vi "Labview.vi"() -> ()   [LabVIEW 2013]
panel:
  out "Array 7":bool[](array[boolean])
  out "Array 6":bool[](array[boolean])
  out "Boolean 7":bool
  out "Boolean 6":bool
  out "Array 5":bool[](array[boolean])
  out "Array 4":bool[](array[boolean])
  out "Array 3":bool[](array[boolean])
  out "Array 2":bool[](array[boolean])
  out "Boolean 5":bool
  out "Boolean 4":bool
  out "Boolean 3":bool
  out "Boolean 2":bool
  out "Boolean":bool
  out "Array 1":bool[](array[boolean])
  in  "string":string
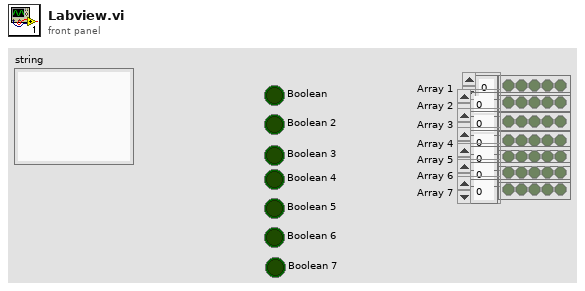
[diagram p1: front panel]
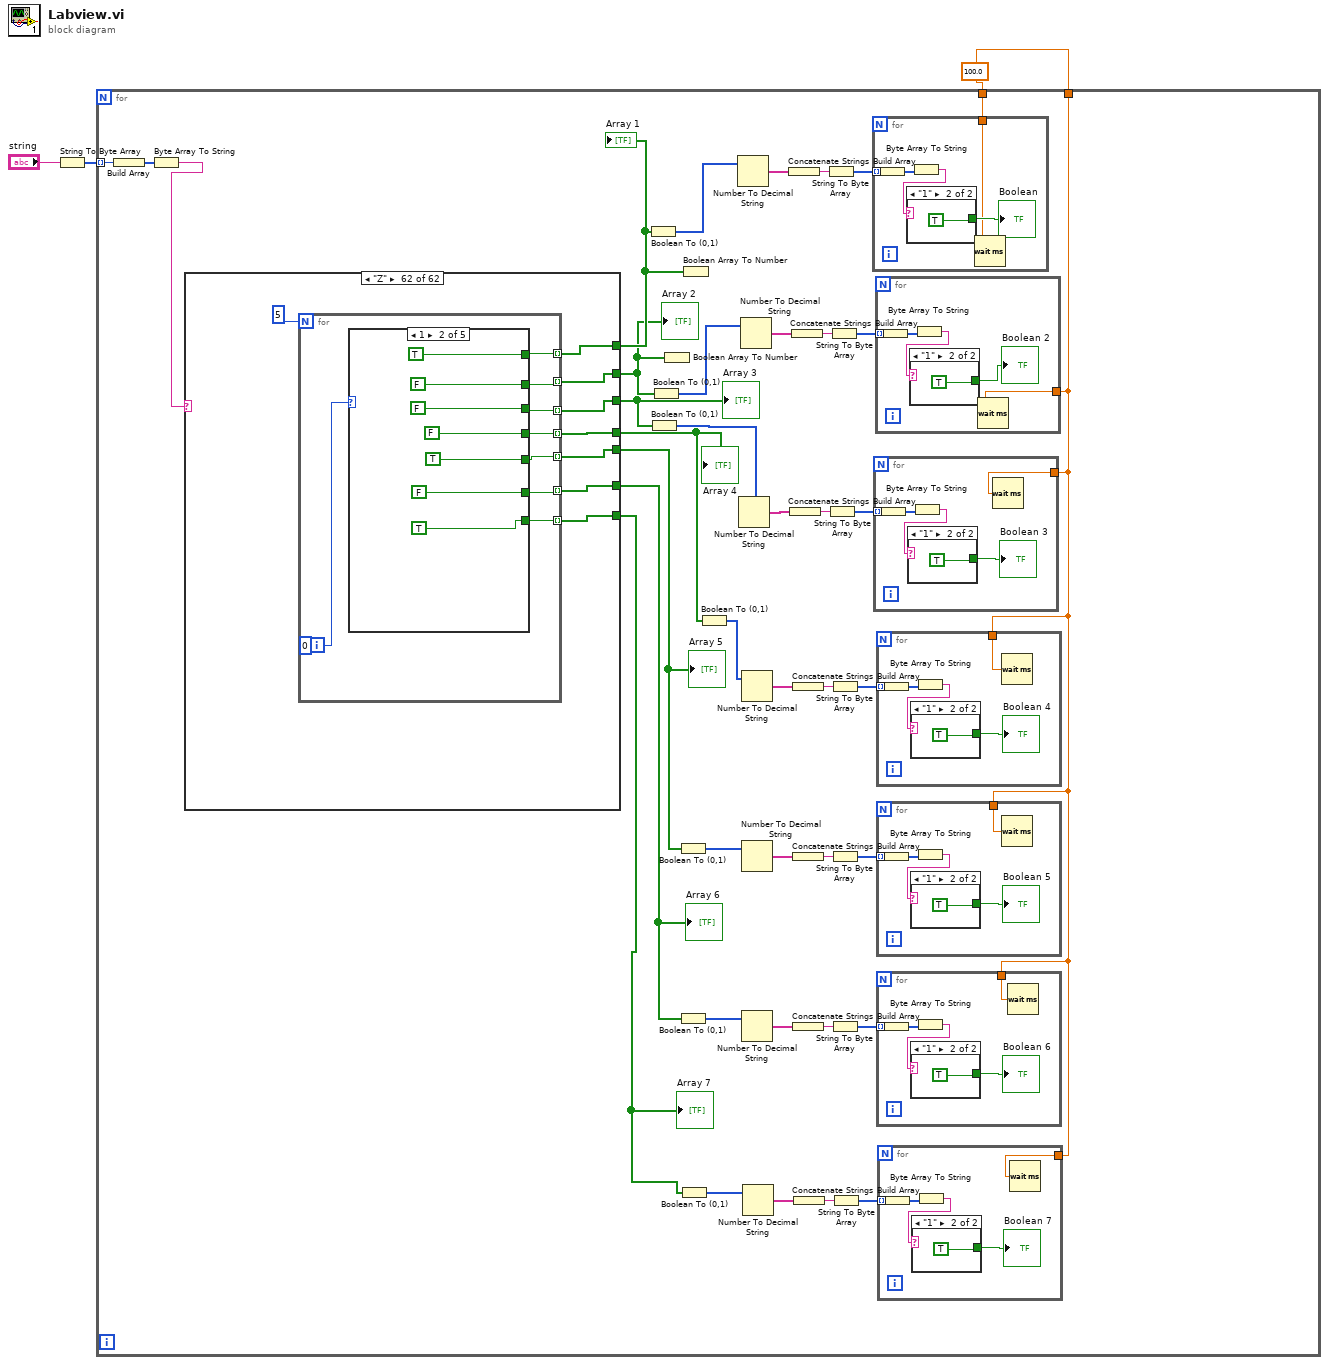
[diagram p0: block diagram]
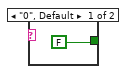
[diagram p2: hidden frame]
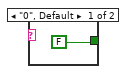
[diagram p3: hidden frame]
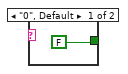
[diagram p4: hidden frame]
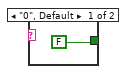
[diagram p5: hidden frame]
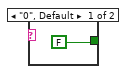
[diagram p6: hidden frame]
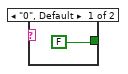
[diagram p7: hidden frame]
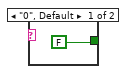
[diagram p8: hidden frame]
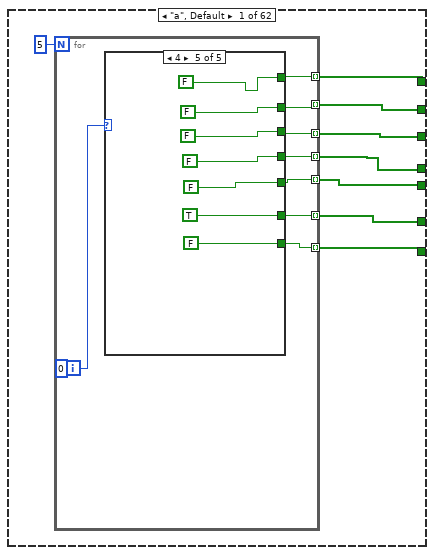
[diagram p9: hidden frame]
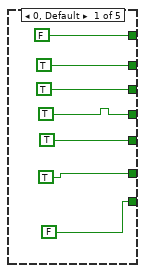
[diagram p10: hidden frame]
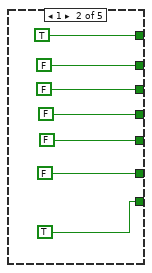
[diagram p11: hidden frame]
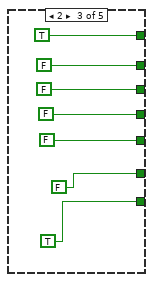
[diagram p12: hidden frame]
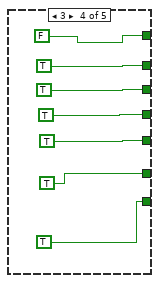
[diagram p13: hidden frame]
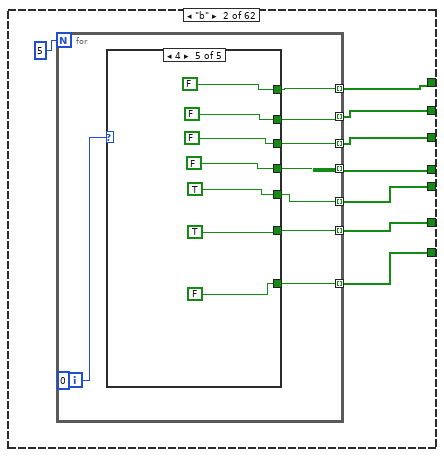
[diagram p14: hidden frame]
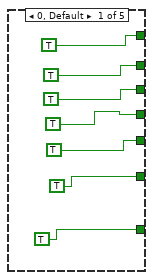
[diagram p15: hidden frame]
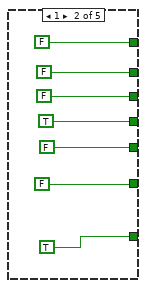
[diagram p16: hidden frame]
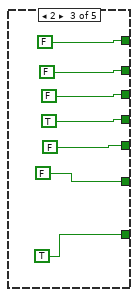
[diagram p17: hidden frame]
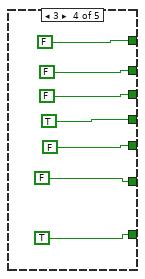
[diagram p18: hidden frame]
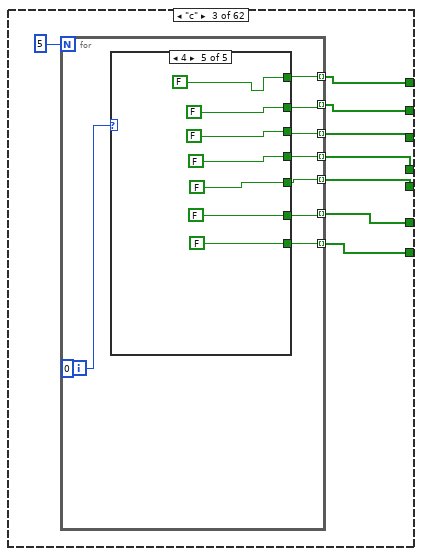
[diagram p19: hidden frame]
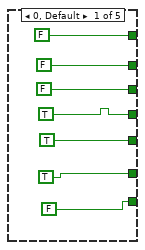
[diagram p20: hidden frame]
diagram:
  w1 = 100.0
  n1 = String To Byte Array(string="string") -> (unsigned byte array=w3:u8[])
  n2 = for {
    tunnel: w3 -> [w43] mode=indexing
    tunnel: w1 -> [w5]
    tunnel: w1 -> [w4]
    n3 = Build Array(w43) -> (w42:u8[])
    n4 = Byte Array To String(unsigned byte array=w42) -> (string=w41:string)
    n5 = case shown="\"Z\"" w41 {
      tunnel: [w99 w146 w201 w252 w303 w354 w405 w456 w507 w558 w609 w660 w711 w762 w813 w864 w915 w966 w1017 w1068 w1119 w1170 w1221 w1272 w1323 w1374 w1425 w1476 w1527 w1578 w1629 w1680 w1731 w1782 w1833 w1884 w1935 w1986 w2037 w2088 w2139 w2190 w2241 w2292 w2343 w2394 w2445 w2496 w2547 w2598 w2649 w2700 w2751 w2802 w2853 w2904 w2955 w3006 w3057 w3108 w3159 w3210] -> w18
      tunnel: [w98 w150 w200 w251 w302 w353 w404 w455 w506 w557 w608 w659 w710 w761 w812 w863 w914 w965 w1016 w1067 w1118 w1169 w1220 w1271 w1322 w1373 w1424 w1475 w1526 w1577 w1628 w1679 w1730 w1781 w1832 w1883 w1934 w1985 w2036 w2087 w2138 w2189 w2240 w2291 w2342 w2393 w2444 w2495 w2546 w2597 w2648 w2699 w2750 w2801 w2852 w2903 w2954 w3005 w3056 w3107 w3158 w3209] -> w17
      tunnel: [w97 w149 w199 w250 w301 w352 w403 w454 w505 w556 w607 w658 w709 w760 w811 w862 w913 w964 w1015 w1066 w1117 w1168 w1219 w1270 w1321 w1372 w1423 w1474 w1525 w1576 w1627 w1678 w1729 w1780 w1831 w1882 w1933 w1984 w2035 w2086 w2137 w2188 w2239 w2290 w2341 w2392 w2443 w2494 w2545 w2596 w2647 w2698 w2749 w2800 w2851 w2902 w2953 w3004 w3055 w3106 w3157 w3208] -> w29
      tunnel: [w96 w148 w198 w249 w300 w351 w402 w453 w504 w555 w606 w657 w708 w759 w810 w861 w912 w963 w1014 w1065 w1116 w1167 w1218 w1269 w1320 w1371 w1422 w1473 w1524 w1575 w1626 w1677 w1728 w1779 w1830 w1881 w1932 w1983 w2034 w2085 w2136 w2187 w2238 w2289 w2340 w2391 w2442 w2493 w2544 w2595 w2646 w2697 w2748 w2799 w2850 w2901 w2952 w3003 w3054 w3105 w3156 w3207] -> w24
      tunnel: [w95 w147 w197 w248 w299 w350 w401 w452 w503 w554 w605 w656 w707 w758 w809 w860 w911 w962 w1013 w1064 w1115 w1166 w1217 w1268 w1319 w1370 w1421 w1472 w1523 w1574 w1625 w1676 w1727 w1778 w1829 w1880 w1931 w1982 w2033 w2084 w2135 w2186 w2237 w2288 w2339 w2390 w2441 w2492 w2543 w2594 w2645 w2696 w2747 w2798 w2849 w2900 w2951 w3002 w3053 w3104 w3155 w3206] -> w16
      tunnel: [w94 w145 w196 w247 w298 w349 w400 w451 w502 w553 w604 w655 w706 w757 w808 w859 w910 w961 w1012 w1063 w1114 w1165 w1216 w1267 w1318 w1369 w1420 w1471 w1522 w1573 w1624 w1675 w1726 w1777 w1828 w1879 w1930 w1981 w2032 w2083 w2134 w2185 w2236 w2287 w2338 w2389 w2440 w2491 w2542 w2593 w2644 w2695 w2746 w2797 w2848 w2899 w2950 w3001 w3052 w3103 w3154 w3205] -> w7
      tunnel: [w93 w144 w195 w246 w297 w348 w399 w450 w501 w552 w603 w654 w705 w756 w807 w858 w909 w960 w1011 w1062 w1113 w1164 w1215 w1266 w1317 w1368 w1419 w1470 w1521 w1572 w1623 w1674 w1725 w1776 w1827 w1878 w1929 w1980 w2031 w2082 w2133 w2184 w2235 w2286 w2337 w2388 w2439 w2490 w2541 w2592 w2643 w2694 w2745 w2796 w2847 w2898 w2949 w3000 w3051 w3102 w3153 w3204] -> w6
      frame "a", Default {
        n6 = for {
          N: 5 -> [_]
          tunnel: [w107] -> w99 mode=indexing
          tunnel: [w106] -> w98 mode=indexing
          tunnel: [w105] -> w97 mode=indexing
          tunnel: [w104] -> w96 mode=indexing
          tunnel: [w103] -> w95 mode=indexing
          tunnel: [w102] -> w94 mode=indexing
          tunnel: [w101] -> w93 mode=indexing
          i -> [w108]
          (unwired) 0
          n7 = case shown="4" w108 {
            tunnel: [FALSE TRUE TRUE FALSE FALSE] -> w107
            tunnel: [TRUE FALSE FALSE TRUE FALSE] -> w106
            tunnel: [TRUE FALSE FALSE TRUE FALSE] -> w105
            tunnel: [TRUE FALSE FALSE TRUE FALSE] -> w104
            tunnel: [TRUE FALSE FALSE TRUE FALSE] -> w103
            tunnel: [TRUE FALSE FALSE TRUE TRUE] -> w102
            tunnel: [FALSE TRUE TRUE TRUE FALSE] -> w101
            frame 0, Default {
            }
            frame 1 {
            }
            frame 2 {
            }
            frame 3 {
            }
            frame 4 {
            }
          }
        }
      }
      frame "b" {
        n8 = for {
          N: 5 -> [_]
          tunnel: [w158] -> w146 mode=indexing
          tunnel: [w157] -> w150 mode=indexing
          tunnel: [w156] -> w149 mode=indexing
          tunnel: [w155] -> w148 mode=indexing
          tunnel: [w154] -> w147 mode=indexing
          tunnel: [w153] -> w145 mode=indexing
          tunnel: [w152] -> w144 mode=indexing
          i -> [w159]
          (unwired) 0
          n9 = case shown="4" w159 {
            tunnel: [TRUE FALSE FALSE FALSE FALSE] -> w158
            tunnel: [TRUE FALSE FALSE FALSE FALSE] -> w157
            tunnel: [TRUE FALSE FALSE FALSE FALSE] -> w156
            tunnel: [TRUE TRUE TRUE TRUE FALSE] -> w155
            tunnel: [TRUE FALSE FALSE FALSE TRUE] -> w154
            tunnel: [TRUE FALSE FALSE FALSE TRUE] -> w153
            tunnel: [TRUE TRUE TRUE TRUE FALSE] -> w152
            frame 0, Default {
            }
            frame 1 {
            }
            frame 2 {
            }
            frame 3 {
            }
            frame 4 {
            }
          }
        }
      }
      frame "c" {
        n10 = for {
          N: 5 -> [_]
          tunnel: [w209] -> w201 mode=indexing
          tunnel: [w208] -> w200 mode=indexing
          tunnel: [w207] -> w199 mode=indexing
          tunnel: [w206] -> w198 mode=indexing
          tunnel: [w205] -> w197 mode=indexing
          tunnel: [w204] -> w196 mode=indexing
          tunnel: [w203] -> w195 mode=indexing
          i -> [w210]
          (unwired) 0
          n11 = case shown="4" w210 {
            tunnel: [FALSE FALSE FALSE FALSE FALSE] -> w209
            tunnel: [FALSE FALSE FALSE FALSE FALSE] -> w208
            tunnel: [FALSE TRUE TRUE FALSE FALSE] -> w207
            tunnel: [TRUE FALSE FALSE TRUE FALSE] -> w206
            tunnel: [TRUE FALSE FALSE FALSE FALSE] -> w205
            tunnel: [TRUE FALSE FALSE FALSE FALSE] -> w204
            tunnel: [FALSE TRUE TRUE TRUE FALSE] -> w203
            frame 0, Default {
            }
            frame 1 {
            }
            frame 2 {
            }
            frame 3 {
            }
            frame 4 {
            }
          }
        }
      }
      frame "d" {
        n12 = for {
          N: 5 -> [_]
          tunnel: [w260] -> w252 mode=indexing
          tunnel: [w259] -> w251 mode=indexing
          tunnel: [w258] -> w250 mode=indexing
          tunnel: [w257] -> w249 mode=indexing
          tunnel: [w256] -> w248 mode=indexing
          tunnel: [w255] -> w247 mode=indexing
          tunnel: [w254] -> w246 mode=indexing
          i -> [w261]
          (unwired) 0
          n13 = case shown="0, Default" w261 {
            tunnel: [FALSE FALSE FALSE FALSE TRUE] -> w260
            tunnel: [FALSE FALSE FALSE FALSE TRUE] -> w259
            tunnel: [FALSE TRUE TRUE TRUE TRUE] -> w258
            tunnel: [TRUE FALSE FALSE FALSE TRUE] -> w257
            tunnel: [TRUE FALSE FALSE FALSE TRUE] -> w256
            tunnel: [TRUE FALSE FALSE FALSE TRUE] -> w255
            tunnel: [FALSE TRUE TRUE TRUE TRUE] -> w254
            frame 0, Default {
            }
            frame 1 {
            }
            frame 2 {
            }
            frame 3 {
            }
            frame 4 {
            }
          }
        }
      }
      frame "e" {
        n14 = for {
          N: 5 -> [_]
          tunnel: [w311] -> w303 mode=indexing
          tunnel: [w310] -> w302 mode=indexing
          tunnel: [w309] -> w301 mode=indexing
          tunnel: [w308] -> w300 mode=indexing
          tunnel: [w307] -> w299 mode=indexing
          tunnel: [w306] -> w298 mode=indexing
          tunnel: [w305] -> w297 mode=indexing
          i -> [w312]
          (unwired) 0
          n15 = case shown="0, Default" w312 {
            tunnel: [FALSE FALSE FALSE FALSE FALSE] -> w311
            tunnel: [FALSE FALSE FALSE FALSE FALSE] -> w310
            tunnel: [FALSE TRUE TRUE TRUE TRUE] -> w309
            tunnel: [TRUE FALSE FALSE FALSE TRUE] -> w308
            tunnel: [TRUE TRUE TRUE TRUE TRUE] -> w307
            tunnel: [TRUE FALSE FALSE FALSE FALSE] -> w306
            tunnel: [FALSE TRUE TRUE TRUE TRUE] -> w305
            frame 0, Default {
            }
            frame 1 {
            }
            frame 2 {
            }
            frame 3 {
            }
            frame 4 {
            }
          }
        }
      }
      frame "f" {
        n16 = for {
          N: 5 -> [_]
          tunnel: [w362] -> w354 mode=indexing
          tunnel: [w361] -> w353 mode=indexing
          tunnel: [w360] -> w352 mode=indexing
          tunnel: [w359] -> w351 mode=indexing
          tunnel: [w358] -> w350 mode=indexing
          tunnel: [w357] -> w349 mode=indexing
          tunnel: [w356] -> w348 mode=indexing
          i -> [w363]
          (unwired) 0
          n17 = case shown="0, Default" w363 {
            tunnel: [FALSE FALSE TRUE TRUE FALSE] -> w362
            tunnel: [FALSE FALSE TRUE FALSE TRUE] -> w361
            tunnel: [FALSE FALSE TRUE FALSE FALSE] -> w360
            tunnel: [FALSE TRUE TRUE TRUE FALSE] -> w359
            tunnel: [FALSE FALSE TRUE FALSE FALSE] -> w358
            tunnel: [FALSE FALSE TRUE FALSE FALSE] -> w357
            tunnel: [FALSE TRUE TRUE FALSE FALSE] -> w356
            frame 0, Default {
            }
            frame 1 {
            }
            frame 2 {
            }
            frame 3 {
            }
            frame 4 {
            }
          }
        }
      }
      frame "g" {
        n18 = for {
          N: 5 -> [_]
          tunnel: [w413] -> w405 mode=indexing
          tunnel: [w412] -> w404 mode=indexing
          tunnel: [w411] -> w403 mode=indexing
          tunnel: [w410] -> w402 mode=indexing
          tunnel: [w409] -> w401 mode=indexing
          tunnel: [w408] -> w400 mode=indexing
          tunnel: [w407] -> w399 mode=indexing
          i -> [w414]
          (unwired) 0
          n19 = case shown="0, Default" w414 {
            tunnel: [FALSE TRUE TRUE TRUE FALSE] -> w413
            tunnel: [TRUE FALSE FALSE FALSE TRUE] -> w412
            tunnel: [TRUE FALSE FALSE FALSE TRUE] -> w411
            tunnel: [FALSE FALSE TRUE TRUE TRUE] -> w410
            tunnel: [FALSE FALSE FALSE FALSE TRUE] -> w409
            tunnel: [TRUE TRUE FALSE TRUE TRUE] -> w408
            tunnel: [FALSE TRUE TRUE TRUE FALSE] -> w407
            frame 0, Default {
            }
            frame 1 {
            }
            frame 2 {
            }
            frame 3 {
            }
            frame 4 {
            }
          }
        }
      }
      frame "h" {
        n20 = for {
          N: 5 -> [_]
          tunnel: [w464] -> w456 mode=indexing
          tunnel: [w463] -> w455 mode=indexing
          tunnel: [w462] -> w454 mode=indexing
          tunnel: [w461] -> w453 mode=indexing
          tunnel: [w460] -> w452 mode=indexing
          tunnel: [w459] -> w451 mode=indexing
          tunnel: [w458] -> w450 mode=indexing
          i -> [w465]
          (unwired) 0
          n21 = case shown="0, Default" w465 {
            tunnel: [TRUE FALSE FALSE FALSE FALSE] -> w464
            tunnel: [TRUE FALSE FALSE FALSE FALSE] -> w463
            tunnel: [TRUE FALSE FALSE FALSE FALSE] -> w462
            tunnel: [TRUE TRUE TRUE TRUE FALSE] -> w461
            tunnel: [TRUE FALSE FALSE FALSE TRUE] -> w460
            tunnel: [TRUE FALSE FALSE FALSE TRUE] -> w459
            tunnel: [TRUE FALSE FALSE FALSE TRUE] -> w458
            frame 0, Default {
            }
            frame 1 {
            }
            frame 2 {
            }
            frame 3 {
            }
            frame 4 {
            }
          }
        }
      }
      frame "i" {
        n22 = for {
          N: 5 -> [_]
          tunnel: [w515] -> w507 mode=indexing
          tunnel: [w514] -> w506 mode=indexing
          tunnel: [w513] -> w505 mode=indexing
          tunnel: [w512] -> w504 mode=indexing
          tunnel: [w511] -> w503 mode=indexing
          tunnel: [w510] -> w502 mode=indexing
          tunnel: [w509] -> w501 mode=indexing
          i -> [w516]
          (unwired) 0
          n23 = case shown="4" w516 {
            tunnel: [FALSE FALSE FALSE FALSE FALSE] -> w515
            tunnel: [FALSE FALSE TRUE FALSE FALSE] -> w514
            tunnel: [FALSE FALSE FALSE FALSE FALSE] -> w513
            tunnel: [FALSE FALSE TRUE FALSE FALSE] -> w512
            tunnel: [FALSE FALSE TRUE FALSE FALSE] -> w511
            tunnel: [FALSE FALSE TRUE FALSE FALSE] -> w510
            tunnel: [FALSE FALSE TRUE FALSE FALSE] -> w509
            frame 0, Default {
            }
            frame 1 {
            }
            frame 2 {
            }
            frame 3 {
            }
            frame 4 {
            }
          }
        }
      }
      frame "j" {
        n24 = for {
          N: 5 -> [_]
          tunnel: [w566] -> w558 mode=indexing
          tunnel: [w565] -> w557 mode=indexing
          tunnel: [w564] -> w556 mode=indexing
          tunnel: [w563] -> w555 mode=indexing
          tunnel: [w562] -> w554 mode=indexing
          tunnel: [w561] -> w553 mode=indexing
          tunnel: [w560] -> w552 mode=indexing
          i -> [w567]
          (unwired) 0
          n25 = case shown="0, Default" w567 {
            tunnel: [FALSE FALSE FALSE FALSE FALSE] -> w566
            tunnel: [FALSE FALSE TRUE FALSE FALSE] -> w565
            tunnel: [FALSE FALSE FALSE FALSE FALSE] -> w564
            tunnel: [FALSE FALSE TRUE FALSE FALSE] -> w563
            tunnel: [FALSE FALSE TRUE FALSE FALSE] -> w562
            tunnel: [TRUE FALSE TRUE FALSE FALSE] -> w561
            tunnel: [FALSE TRUE TRUE FALSE FALSE] -> w560
            frame 0, Default {
            }
            frame 1 {
            }
            frame 2 {
            }
            frame 3 {
            }
            frame 4 {
            }
          }
        }
      }
      frame "k" {
        n26 = for {
          N: 5 -> [_]
          tunnel: [w617] -> w609 mode=indexing
          tunnel: [w616] -> w608 mode=indexing
          tunnel: [w615] -> w607 mode=indexing
          tunnel: [w614] -> w606 mode=indexing
          tunnel: [w613] -> w605 mode=indexing
          tunnel: [w612] -> w604 mode=indexing
          tunnel: [w611] -> w603 mode=indexing
          i -> [w618]
          (unwired) 0
          n27 = case shown="0, Default" w618 {
            tunnel: [TRUE FALSE FALSE FALSE FALSE] -> w617
            tunnel: [TRUE FALSE FALSE FALSE FALSE] -> w616
            tunnel: [TRUE FALSE FALSE TRUE FALSE] -> w615
            tunnel: [TRUE FALSE TRUE FALSE FALSE] -> w614
            tunnel: [TRUE TRUE FALSE FALSE FALSE] -> w613
            tunnel: [TRUE FALSE TRUE FALSE FALSE] -> w612
            tunnel: [TRUE FALSE FALSE TRUE FALSE] -> w611
            frame 0, Default {
            }
            frame 1 {
            }
            frame 2 {
            }
            frame 3 {
            }
            frame 4 {
            }
          }
        }
      }
      frame "l" {
        n28 = for {
          N: 5 -> [_]
          tunnel: [w668] -> w660 mode=indexing
          tunnel: [w667] -> w659 mode=indexing
          tunnel: [w666] -> w658 mode=indexing
          tunnel: [w665] -> w657 mode=indexing
          tunnel: [w664] -> w656 mode=indexing
          tunnel: [w663] -> w655 mode=indexing
          tunnel: [w662] -> w654 mode=indexing
          i -> [w669]
          (unwired) 0
          n29 = case shown="4" w669 {
            tunnel: [FALSE FALSE TRUE FALSE FALSE] -> w668
            tunnel: [FALSE FALSE TRUE FALSE FALSE] -> w667
            tunnel: [TRUE FALSE TRUE FALSE FALSE] -> w666
            tunnel: [TRUE FALSE TRUE FALSE FALSE] -> w665
            tunnel: [TRUE FALSE TRUE FALSE FALSE] -> w664
            tunnel: [TRUE FALSE TRUE FALSE FALSE] -> w663
            tunnel: [TRUE FALSE TRUE FALSE FALSE] -> w662
            frame 0, Default {
            }
            frame 1 {
            }
            frame 2 {
            }
            frame 3 {
            }
            frame 4 {
            }
          }
        }
      }
      frame "m" {
        n30 = for {
          N: 5 -> [_]
          tunnel: [w719] -> w711 mode=indexing
          tunnel: [w718] -> w710 mode=indexing
          tunnel: [w717] -> w709 mode=indexing
          tunnel: [w716] -> w708 mode=indexing
          tunnel: [w715] -> w707 mode=indexing
          tunnel: [w714] -> w706 mode=indexing
          tunnel: [w713] -> w705 mode=indexing
          i -> [w720]
          (unwired) 0
          n31 = case shown="4" w720 {
            tunnel: [FALSE FALSE FALSE FALSE FALSE] -> w719
            tunnel: [FALSE FALSE FALSE FALSE FALSE] -> w718
            tunnel: [FALSE FALSE FALSE FALSE FALSE] -> w717
            tunnel: [FALSE TRUE FALSE FALSE TRUE] -> w716
            tunnel: [TRUE FALSE TRUE FALSE TRUE] -> w715
            tunnel: [TRUE FALSE TRUE FALSE TRUE] -> w714
            tunnel: [TRUE FALSE TRUE FALSE TRUE] -> w713
            frame 0, Default {
            }
            frame 1 {
            }
            frame 2 {
            }
            frame 3 {
            }
            frame 4 {
            }
          }
        }
      }
      frame "n" {
        n32 = for {
          N: 5 -> [_]
          tunnel: [w770] -> w762 mode=indexing
          tunnel: [w769] -> w761 mode=indexing
          tunnel: [w768] -> w760 mode=indexing
          tunnel: [w767] -> w759 mode=indexing
          tunnel: [w766] -> w758 mode=indexing
          tunnel: [w765] -> w757 mode=indexing
          tunnel: [w764] -> w756 mode=indexing
          i -> [w771]
          (unwired) 0
          n33 = case shown="4" w771 {
            tunnel: [FALSE FALSE FALSE FALSE FALSE] -> w770
            tunnel: [FALSE FALSE FALSE FALSE FALSE] -> w769
            tunnel: [FALSE FALSE FALSE FALSE FALSE] -> w768
            tunnel: [TRUE FALSE TRUE TRUE FALSE] -> w767
            tunnel: [FALSE TRUE FALSE FALSE TRUE] -> w766
            tunnel: [FALSE TRUE FALSE FALSE TRUE] -> w765
            tunnel: [FALSE TRUE FALSE FALSE TRUE] -> w764
            frame 0, Default {
            }
            frame 1 {
            }
            frame 2 {
            }
            frame 3 {
            }
            frame 4 {
            }
          }
        }
      }
      frame "o" {
        n34 = for {
          N: 5 -> [_]
          tunnel: [w821] -> w813 mode=indexing
          tunnel: [w820] -> w812 mode=indexing
          tunnel: [w819] -> w811 mode=indexing
          tunnel: [w818] -> w810 mode=indexing
          tunnel: [w817] -> w809 mode=indexing
          tunnel: [w816] -> w808 mode=indexing
          tunnel: [w815] -> w807 mode=indexing
          i -> [w822]
          (unwired) 0
          n35 = case shown="0, Default" w822 {
            tunnel: [FALSE FALSE FALSE FALSE FALSE] -> w821
            tunnel: [FALSE FALSE FALSE FALSE FALSE] -> w820
            tunnel: [FALSE TRUE TRUE TRUE FALSE] -> w819
            tunnel: [TRUE FALSE FALSE FALSE TRUE] -> w818
            tunnel: [TRUE FALSE FALSE FALSE TRUE] -> w817
            tunnel: [TRUE FALSE FALSE FALSE TRUE] -> w816
            tunnel: [FALSE TRUE TRUE TRUE FALSE] -> w815
            frame 0, Default {
            }
            frame 1 {
            }
            frame 2 {
            }
            frame 3 {
            }
            frame 4 {
            }
          }
        }
      }
      frame "p" {
        n36 = for {
          N: 5 -> [_]
          tunnel: [w872] -> w864 mode=indexing
          tunnel: [w871] -> w863 mode=indexing
          tunnel: [w870] -> w862 mode=indexing
          tunnel: [w869] -> w861 mode=indexing
          tunnel: [w868] -> w860 mode=indexing
          tunnel: [w867] -> w859 mode=indexing
          tunnel: [w866] -> w858 mode=indexing
          i -> [w873]
          (unwired) 0
          n37 = case shown="4" w873 {
            tunnel: [TRUE FALSE FALSE FALSE FALSE] -> w872
            tunnel: [TRUE TRUE TRUE FALSE FALSE] -> w871
            tunnel: [TRUE FALSE FALSE TRUE FALSE] -> w870
            tunnel: [TRUE TRUE TRUE FALSE FALSE] -> w869
            tunnel: [TRUE FALSE FALSE FALSE FALSE] -> w868
            tunnel: [TRUE FALSE FALSE FALSE FALSE] -> w867
            tunnel: [TRUE FALSE FALSE FALSE FALSE] -> w866
            frame 0, Default {
            }
            frame 1 {
            }
            frame 2 {
            }
            frame 3 {
            }
            frame 4 {
            }
          }
        }
      }
      frame "q" {
        n38 = for {
          N: 5 -> [_]
          tunnel: [w923] -> w915 mode=indexing
          tunnel: [w922] -> w914 mode=indexing
          tunnel: [w921] -> w913 mode=indexing
          tunnel: [w920] -> w912 mode=indexing
          tunnel: [w919] -> w911 mode=indexing
          tunnel: [w918] -> w910 mode=indexing
          tunnel: [w917] -> w909 mode=indexing
          i -> [w924]
          (unwired) 0
          n39 = case shown="4" w924 {
            tunnel: [FALSE TRUE TRUE FALSE FALSE] -> w923
            tunnel: [TRUE FALSE FALSE TRUE FALSE] -> w922
            tunnel: [TRUE FALSE FALSE TRUE FALSE] -> w921
            tunnel: [TRUE TRUE TRUE TRUE FALSE] -> w920
            tunnel: [FALSE FALSE FALSE FALSE FALSE] -> w919
            tunnel: [FALSE FALSE FALSE TRUE TRUE] -> w918
            tunnel: [FALSE FALSE FALSE TRUE FALSE] -> w917
            frame 0, Default {
            }
            frame 1 {
            }
            frame 2 {
            }
            frame 3 {
            }
            frame 4 {
            }
          }
        }
      }
      frame "r" {
        n40 = for {
          N: 5 -> [_]
          tunnel: [w974] -> w966 mode=indexing
          tunnel: [w973] -> w965 mode=indexing
          tunnel: [w972] -> w964 mode=indexing
          tunnel: [w971] -> w963 mode=indexing
          tunnel: [w970] -> w962 mode=indexing
          tunnel: [w969] -> w961 mode=indexing
          tunnel: [w968] -> w960 mode=indexing
          i -> [w975]
          (unwired) 0
          n41 = case shown="4" w975 {
            tunnel: [FALSE FALSE FALSE FALSE FALSE] -> w974
            tunnel: [FALSE TRUE FALSE TRUE TRUE] -> w973
            tunnel: [FALSE FALSE TRUE FALSE FALSE] -> w972
            tunnel: [FALSE FALSE TRUE FALSE FALSE] -> w971
            tunnel: [FALSE FALSE TRUE FALSE FALSE] -> w970
            tunnel: [FALSE FALSE TRUE FALSE FALSE] -> w969
            tunnel: [FALSE TRUE TRUE FALSE FALSE] -> w968
            frame 0, Default {
            }
            frame 1 {
            }
            frame 2 {
            }
            frame 3 {
            }
            frame 4 {
            }
          }
        }
      }
      frame "s" {
        n42 = for {
          N: 5 -> [_]
          tunnel: [w1025] -> w1017 mode=indexing
          tunnel: [w1024] -> w1016 mode=indexing
          tunnel: [w1023] -> w1015 mode=indexing
          tunnel: [w1022] -> w1014 mode=indexing
          tunnel: [w1021] -> w1013 mode=indexing
          tunnel: [w1020] -> w1012 mode=indexing
          tunnel: [w1019] -> w1011 mode=indexing
          i -> [w1026]
          (unwired) 0
          n43 = case shown="4" w1026 {
            tunnel: [FALSE FALSE FALSE FALSE FALSE] -> w1025
            tunnel: [FALSE FALSE FALSE FALSE FALSE] -> w1024
            tunnel: [FALSE TRUE TRUE TRUE TRUE] -> w1023
            tunnel: [TRUE FALSE FALSE FALSE FALSE] -> w1022
            tunnel: [TRUE TRUE TRUE TRUE TRUE] -> w1021
            tunnel: [FALSE FALSE FALSE FALSE TRUE] -> w1020
            tunnel: [TRUE TRUE TRUE TRUE FALSE] -> w1019
            frame 0, Default {
            }
            frame 1 {
            }
            frame 2 {
            }
            frame 3 {
            }
            frame 4 {
            }
          }
        }
      }
      frame "t" {
        n44 = for {
          N: 5 -> [_]
          tunnel: [w1076] -> w1068 mode=indexing
          tunnel: [w1075] -> w1067 mode=indexing
          tunnel: [w1074] -> w1066 mode=indexing
          tunnel: [w1073] -> w1065 mode=indexing
          tunnel: [w1072] -> w1064 mode=indexing
          tunnel: [w1071] -> w1063 mode=indexing
          tunnel: [w1070] -> w1062 mode=indexing
          i -> [w1077]
          (unwired) 0
          n45 = case shown="4" w1077 {
            tunnel: [FALSE FALSE TRUE FALSE FALSE] -> w1076
            tunnel: [FALSE FALSE TRUE FALSE FALSE] -> w1075
            tunnel: [FALSE TRUE TRUE TRUE FALSE] -> w1074
            tunnel: [FALSE FALSE TRUE FALSE FALSE] -> w1073
            tunnel: [FALSE FALSE TRUE FALSE FALSE] -> w1072
            tunnel: [FALSE FALSE TRUE FALSE TRUE] -> w1071
            tunnel: [FALSE FALSE TRUE TRUE FALSE] -> w1070
            frame 0, Default {
            }
            frame 1 {
            }
            frame 2 {
            }
            frame 3 {
            }
            frame 4 {
            }
          }
        }
      }
      frame "u" {
        n46 = for {
          N: 5 -> [_]
          tunnel: [w1127] -> w1119 mode=indexing
          tunnel: [w1126] -> w1118 mode=indexing
          tunnel: [w1125] -> w1117 mode=indexing
          tunnel: [w1124] -> w1116 mode=indexing
          tunnel: [w1123] -> w1115 mode=indexing
          tunnel: [w1122] -> w1114 mode=indexing
          tunnel: [w1121] -> w1113 mode=indexing
          i -> [w1128]
          (unwired) 0
          n47 = case shown="4" w1128 {
            tunnel: [FALSE FALSE FALSE FALSE FALSE] -> w1127
            tunnel: [FALSE FALSE FALSE FALSE FALSE] -> w1126
            tunnel: [TRUE FALSE FALSE FALSE TRUE] -> w1125
            tunnel: [TRUE FALSE FALSE FALSE TRUE] -> w1124
            tunnel: [TRUE FALSE FALSE FALSE TRUE] -> w1123
            tunnel: [TRUE FALSE FALSE FALSE TRUE] -> w1122
            tunnel: [FALSE TRUE TRUE TRUE TRUE] -> w1121
            frame 0, Default {
            }
            frame 1 {
            }
            frame 2 {
            }
            frame 3 {
            }
            frame 4 {
            }
          }
        }
      }
      frame "v" {
        n48 = for {
          N: 5 -> [_]
          tunnel: [w1178] -> w1170 mode=indexing
          tunnel: [w1177] -> w1169 mode=indexing
          tunnel: [w1176] -> w1168 mode=indexing
          tunnel: [w1175] -> w1167 mode=indexing
          tunnel: [w1174] -> w1166 mode=indexing
          tunnel: [w1173] -> w1165 mode=indexing
          tunnel: [w1172] -> w1164 mode=indexing
          i -> [w1179]
          (unwired) 0
          n49 = case shown="0, Default" w1179 {
            tunnel: [FALSE FALSE FALSE FALSE FALSE] -> w1178
            tunnel: [FALSE FALSE FALSE FALSE FALSE] -> w1177
            tunnel: [TRUE FALSE FALSE FALSE TRUE] -> w1176
            tunnel: [TRUE FALSE FALSE FALSE TRUE] -> w1175
            tunnel: [TRUE FALSE FALSE FALSE TRUE] -> w1174
            tunnel: [FALSE TRUE FALSE TRUE FALSE] -> w1173
            tunnel: [FALSE FALSE TRUE FALSE FALSE] -> w1172
            frame 0, Default {
            }
            frame 1 {
            }
            frame 2 {
            }
            frame 3 {
            }
            frame 4 {
            }
          }
        }
      }
      frame "w" {
        n50 = for {
          N: 5 -> [_]
          tunnel: [w1229] -> w1221 mode=indexing
          tunnel: [w1228] -> w1220 mode=indexing
          tunnel: [w1227] -> w1219 mode=indexing
          tunnel: [w1226] -> w1218 mode=indexing
          tunnel: [w1225] -> w1217 mode=indexing
          tunnel: [w1224] -> w1216 mode=indexing
          tunnel: [w1223] -> w1215 mode=indexing
          i -> [w1230]
          (unwired) 0
          n51 = case shown="2" w1230 {
            tunnel: [FALSE FALSE FALSE FALSE FALSE] -> w1229
            tunnel: [FALSE FALSE FALSE FALSE FALSE] -> w1228
            tunnel: [FALSE FALSE FALSE FALSE FALSE] -> w1227
            tunnel: [TRUE FALSE TRUE FALSE TRUE] -> w1226
            tunnel: [TRUE FALSE TRUE FALSE TRUE] -> w1225
            tunnel: [TRUE FALSE TRUE FALSE TRUE] -> w1224
            tunnel: [FALSE TRUE FALSE TRUE FALSE] -> w1223
            frame 0, Default {
            }
            frame 1 {
            }
            frame 2 {
            }
            frame 3 {
            }
            frame 4 {
            }
          }
        }
      }
      frame "x" {
        n52 = for {
          N: 5 -> [_]
          tunnel: [w1280] -> w1272 mode=indexing
          tunnel: [w1279] -> w1271 mode=indexing
          tunnel: [w1278] -> w1270 mode=indexing
          tunnel: [w1277] -> w1269 mode=indexing
          tunnel: [w1276] -> w1268 mode=indexing
          tunnel: [w1275] -> w1267 mode=indexing
          tunnel: [w1274] -> w1266 mode=indexing
          i -> [w1281]
          (unwired) 0
          n53 = case shown="0, Default" w1281 {
            tunnel: [FALSE FALSE FALSE FALSE FALSE] -> w1280
            tunnel: [FALSE FALSE FALSE FALSE FALSE] -> w1279
            tunnel: [TRUE FALSE FALSE FALSE TRUE] -> w1278
            tunnel: [FALSE TRUE FALSE TRUE FALSE] -> w1277
            tunnel: [FALSE FALSE TRUE FALSE FALSE] -> w1276
            tunnel: [FALSE TRUE FALSE TRUE FALSE] -> w1275
            tunnel: [TRUE FALSE FALSE FALSE TRUE] -> w1274
            frame 0, Default {
            }
            frame 1 {
            }
            frame 2 {
            }
            frame 3 {
            }
            frame 4 {
            }
          }
        }
      }
      frame "y" {
        n54 = for {
          N: 5 -> [_]
          tunnel: [w1331] -> w1323 mode=indexing
          tunnel: [w1330] -> w1322 mode=indexing
          tunnel: [w1329] -> w1321 mode=indexing
          tunnel: [w1328] -> w1320 mode=indexing
          tunnel: [w1327] -> w1319 mode=indexing
          tunnel: [w1326] -> w1318 mode=indexing
          tunnel: [w1325] -> w1317 mode=indexing
          i -> [w1332]
          (unwired) 0
          n55 = case shown="0, Default" w1332 {
            tunnel: [FALSE FALSE FALSE FALSE FALSE] -> w1331
            tunnel: [FALSE FALSE FALSE FALSE FALSE] -> w1330
            tunnel: [TRUE FALSE FALSE FALSE TRUE] -> w1329
            tunnel: [FALSE TRUE FALSE TRUE FALSE] -> w1328
            tunnel: [FALSE FALSE TRUE FALSE FALSE] -> w1327
            tunnel: [FALSE FALSE TRUE FALSE FALSE] -> w1326
            tunnel: [FALSE FALSE TRUE FALSE FALSE] -> w1325
            frame 0, Default {
            }
            frame 1 {
            }
            frame 2 {
            }
            frame 3 {
            }
            frame 4 {
            }
          }
        }
      }
      frame "z" {
        n56 = for {
          N: 5 -> [_]
          tunnel: [w1382] -> w1374 mode=indexing
          tunnel: [w1381] -> w1373 mode=indexing
          tunnel: [w1380] -> w1372 mode=indexing
          tunnel: [w1379] -> w1371 mode=indexing
          tunnel: [w1378] -> w1370 mode=indexing
          tunnel: [w1377] -> w1369 mode=indexing
          tunnel: [w1376] -> w1368 mode=indexing
          i -> [w1383]
          (unwired) 0
          n57 = case shown="3" w1383 {
            tunnel: [FALSE FALSE FALSE FALSE FALSE] -> w1382
            tunnel: [FALSE FALSE FALSE FALSE FALSE] -> w1381
            tunnel: [TRUE TRUE TRUE TRUE TRUE] -> w1380
            tunnel: [FALSE FALSE FALSE TRUE FALSE] -> w1379
            tunnel: [FALSE FALSE TRUE FALSE FALSE] -> w1378
            tunnel: [FALSE TRUE FALSE FALSE FALSE] -> w1377
            tunnel: [TRUE TRUE TRUE TRUE TRUE] -> w1376
            frame 0, Default {
            }
            frame 1 {
            }
            frame 2 {
            }
            frame 3 {
            }
            frame 4 {
            }
          }
        }
      }
      frame "1" {
        n58 = for {
          N: 5 -> [_]
          tunnel: [w1433] -> w1425 mode=indexing
          tunnel: [w1432] -> w1424 mode=indexing
          tunnel: [w1431] -> w1423 mode=indexing
          tunnel: [w1430] -> w1422 mode=indexing
          tunnel: [w1429] -> w1421 mode=indexing
          tunnel: [w1428] -> w1420 mode=indexing
          tunnel: [w1427] -> w1419 mode=indexing
          i -> [w1434]
          (unwired) 0
          n59 = case shown="4" w1434 {
            tunnel: [FALSE FALSE TRUE FALSE FALSE] -> w1433
            tunnel: [FALSE TRUE TRUE FALSE FALSE] -> w1432
            tunnel: [FALSE FALSE TRUE FALSE FALSE] -> w1431
            tunnel: [FALSE FALSE TRUE FALSE FALSE] -> w1430
            tunnel: [FALSE FALSE TRUE FALSE FALSE] -> w1429
            tunnel: [FALSE FALSE TRUE FALSE FALSE] -> w1428
            tunnel: [TRUE TRUE TRUE TRUE TRUE] -> w1427
            frame 0, Default {
            }
            frame 1 {
            }
            frame 2 {
            }
            frame 3 {
            }
            frame 4 {
            }
          }
        }
      }
      frame "2" {
        n60 = for {
          N: 5 -> [_]
          tunnel: [w1484] -> w1476 mode=indexing
          tunnel: [w1483] -> w1475 mode=indexing
          tunnel: [w1482] -> w1474 mode=indexing
          tunnel: [w1481] -> w1473 mode=indexing
          tunnel: [w1480] -> w1472 mode=indexing
          tunnel: [w1479] -> w1471 mode=indexing
          tunnel: [w1478] -> w1470 mode=indexing
          i -> [w1485]
          (unwired) 0
          n61 = case shown="0, Default" w1485 {
            tunnel: [FALSE TRUE TRUE TRUE FALSE] -> w1484
            tunnel: [TRUE FALSE FALSE FALSE TRUE] -> w1483
            tunnel: [FALSE FALSE FALSE TRUE TRUE] -> w1482
            tunnel: [FALSE FALSE TRUE TRUE FALSE] -> w1481
            tunnel: [FALSE TRUE TRUE FALSE FALSE] -> w1480
            tunnel: [TRUE TRUE FALSE FALSE FALSE] -> w1479
            tunnel: [TRUE TRUE TRUE TRUE TRUE] -> w1478
            frame 0, Default {
            }
            frame 1 {
            }
            frame 2 {
            }
            frame 3 {
            }
            frame 4 {
            }
          }
        }
      }
      frame "3" {
        n62 = for {
          N: 5 -> [_]
          tunnel: [w1535] -> w1527 mode=indexing
          tunnel: [w1534] -> w1526 mode=indexing
          tunnel: [w1533] -> w1525 mode=indexing
          tunnel: [w1532] -> w1524 mode=indexing
          tunnel: [w1531] -> w1523 mode=indexing
          tunnel: [w1530] -> w1522 mode=indexing
          tunnel: [w1529] -> w1521 mode=indexing
          i -> [w1536]
          (unwired) 0
          n63 = case shown="0, Default" w1536 {
            tunnel: [TRUE TRUE TRUE TRUE FALSE] -> w1535
            tunnel: [FALSE FALSE FALSE FALSE TRUE] -> w1534
            tunnel: [FALSE FALSE FALSE FALSE TRUE] -> w1533
            tunnel: [FALSE TRUE TRUE TRUE FALSE] -> w1532
            tunnel: [FALSE FALSE FALSE FALSE TRUE] -> w1531
            tunnel: [FALSE FALSE FALSE FALSE TRUE] -> w1530
            tunnel: [TRUE TRUE TRUE TRUE FALSE] -> w1529
            frame 0, Default {
            }
            frame 1 {
            }
            frame 2 {
            }
            frame 3 {
            }
            frame 4 {
            }
          }
        }
      }
      frame "4" {
        n64 = for {
          N: 5 -> [_]
          tunnel: [w1586] -> w1578 mode=indexing
          tunnel: [w1585] -> w1577 mode=indexing
          tunnel: [w1584] -> w1576 mode=indexing
          tunnel: [w1583] -> w1575 mode=indexing
          tunnel: [w1582] -> w1574 mode=indexing
          tunnel: [w1581] -> w1573 mode=indexing
          tunnel: [w1580] -> w1572 mode=indexing
          i -> [w1587]
          (unwired) 0
          n65 = case shown="3" w1587 {
            tunnel: [TRUE FALSE FALSE FALSE FALSE] -> w1586
            tunnel: [TRUE FALSE FALSE FALSE FALSE] -> w1585
            tunnel: [TRUE FALSE FALSE FALSE TRUE] -> w1584
            tunnel: [TRUE FALSE FALSE FALSE TRUE] -> w1583
            tunnel: [TRUE TRUE TRUE TRUE TRUE] -> w1582
            tunnel: [FALSE FALSE FALSE FALSE TRUE] -> w1581
            tunnel: [FALSE FALSE FALSE FALSE TRUE] -> w1580
            frame 0, Default {
            }
            frame 1 {
            }
            frame 2 {
            }
            frame 3 {
            }
            frame 4 {
            }
          }
        }
      }
      frame "5" {
        n66 = for {
          N: 5 -> [_]
          tunnel: [w1637] -> w1629 mode=indexing
          tunnel: [w1636] -> w1628 mode=indexing
          tunnel: [w1635] -> w1627 mode=indexing
          tunnel: [w1634] -> w1626 mode=indexing
          tunnel: [w1633] -> w1625 mode=indexing
          tunnel: [w1632] -> w1624 mode=indexing
          tunnel: [w1631] -> w1623 mode=indexing
          i -> [w1638]
          (unwired) 0
          n67 = case shown="4" w1638 {
            tunnel: [TRUE TRUE TRUE TRUE TRUE] -> w1637
            tunnel: [TRUE FALSE FALSE FALSE FALSE] -> w1636
            tunnel: [TRUE FALSE FALSE FALSE FALSE] -> w1635
            tunnel: [TRUE TRUE TRUE TRUE TRUE] -> w1634
            tunnel: [FALSE FALSE FALSE FALSE TRUE] -> w1633
            tunnel: [TRUE FALSE FALSE FALSE TRUE] -> w1632
            tunnel: [FALSE TRUE TRUE TRUE FALSE] -> w1631
            frame 0, Default {
            }
            frame 1 {
            }
            frame 2 {
            }
            frame 3 {
            }
            frame 4 {
            }
          }
        }
      }
      frame "6" {
        n68 = for {
          N: 5 -> [_]
          tunnel: [w1688] -> w1680 mode=indexing
          tunnel: [w1687] -> w1679 mode=indexing
          tunnel: [w1686] -> w1678 mode=indexing
          tunnel: [w1685] -> w1677 mode=indexing
          tunnel: [w1684] -> w1676 mode=indexing
          tunnel: [w1683] -> w1675 mode=indexing
          tunnel: [w1682] -> w1674 mode=indexing
          i -> [w1689]
          (unwired) 0
          n69 = case shown="4" w1689 {
            tunnel: [FALSE FALSE FALSE TRUE TRUE] -> w1688
            tunnel: [FALSE TRUE TRUE FALSE FALSE] -> w1687
            tunnel: [TRUE TRUE FALSE FALSE FALSE] -> w1686
            tunnel: [TRUE TRUE TRUE TRUE FALSE] -> w1685
            tunnel: [TRUE FALSE FALSE FALSE TRUE] -> w1684
            tunnel: [TRUE FALSE FALSE FALSE TRUE] -> w1683
            tunnel: [FALSE TRUE TRUE TRUE FALSE] -> w1682
            frame 0, Default {
            }
            frame 1 {
            }
            frame 2 {
            }
            frame 3 {
            }
            frame 4 {
            }
          }
        }
      }
      frame "7" {
        n70 = for {
          N: 5 -> [_]
          tunnel: [w1739] -> w1731 mode=indexing
          tunnel: [w1738] -> w1730 mode=indexing
          tunnel: [w1737] -> w1729 mode=indexing
          tunnel: [w1736] -> w1728 mode=indexing
          tunnel: [w1735] -> w1727 mode=indexing
          tunnel: [w1734] -> w1726 mode=indexing
          tunnel: [w1733] -> w1725 mode=indexing
          i -> [w1740]
          (unwired) 0
          n71 = case shown="2" w1740 {
            tunnel: [TRUE TRUE TRUE TRUE TRUE] -> w1739
            tunnel: [FALSE FALSE FALSE FALSE TRUE] -> w1738
            tunnel: [FALSE FALSE FALSE FALSE TRUE] -> w1737
            tunnel: [FALSE FALSE FALSE FALSE TRUE] -> w1736
            tunnel: [FALSE FALSE FALSE FALSE TRUE] -> w1735
            tunnel: [FALSE FALSE FALSE FALSE TRUE] -> w1734
            tunnel: [FALSE FALSE FALSE FALSE TRUE] -> w1733
            frame 0, Default {
            }
            frame 1 {
            }
            frame 2 {
            }
            frame 3 {
            }
            frame 4 {
            }
          }
        }
      }
      frame "8" {
        n72 = for {
          N: 5 -> [_]
          tunnel: [w1790] -> w1782 mode=indexing
          tunnel: [w1789] -> w1781 mode=indexing
          tunnel: [w1788] -> w1780 mode=indexing
          tunnel: [w1787] -> w1779 mode=indexing
          tunnel: [w1786] -> w1778 mode=indexing
          tunnel: [w1785] -> w1777 mode=indexing
          tunnel: [w1784] -> w1776 mode=indexing
          i -> [w1791]
          (unwired) 0
          n73 = case shown="0, Default" w1791 {
            tunnel: [TRUE TRUE TRUE TRUE TRUE] -> w1790
            tunnel: [TRUE FALSE FALSE FALSE TRUE] -> w1789
            tunnel: [TRUE FALSE FALSE FALSE TRUE] -> w1788
            tunnel: [TRUE TRUE TRUE TRUE TRUE] -> w1787
            tunnel: [TRUE FALSE FALSE FALSE TRUE] -> w1786
            tunnel: [TRUE FALSE FALSE FALSE TRUE] -> w1785
            tunnel: [TRUE TRUE TRUE TRUE TRUE] -> w1784
            frame 0, Default {
            }
            frame 1 {
            }
            frame 2 {
            }
            frame 3 {
            }
            frame 4 {
            }
          }
        }
      }
      frame "9" {
        n74 = for {
          N: 5 -> [_]
          tunnel: [w1841] -> w1833 mode=indexing
          tunnel: [w1840] -> w1832 mode=indexing
          tunnel: [w1839] -> w1831 mode=indexing
          tunnel: [w1838] -> w1830 mode=indexing
          tunnel: [w1837] -> w1829 mode=indexing
          tunnel: [w1836] -> w1828 mode=indexing
          tunnel: [w1835] -> w1827 mode=indexing
          i -> [w1842]
          (unwired) 0
          n75 = case shown="0, Default" w1842 {
            tunnel: [TRUE TRUE TRUE TRUE TRUE] -> w1841
            tunnel: [TRUE FALSE FALSE FALSE TRUE] -> w1840
            tunnel: [TRUE FALSE FALSE FALSE TRUE] -> w1839
            tunnel: [TRUE TRUE TRUE TRUE TRUE] -> w1838
            tunnel: [FALSE FALSE FALSE FALSE TRUE] -> w1837
            tunnel: [FALSE FALSE FALSE FALSE TRUE] -> w1836
            tunnel: [FALSE FALSE FALSE FALSE TRUE] -> w1835
            frame 0, Default {
            }
            frame 1 {
            }
            frame 2 {
            }
            frame 3 {
            }
            frame 4 {
            }
          }
        }
      }
      frame "0" {
        n76 = for {
          N: 5 -> [_]
          tunnel: [w1892] -> w1884 mode=indexing
          tunnel: [w1891] -> w1883 mode=indexing
          tunnel: [w1890] -> w1882 mode=indexing
          tunnel: [w1889] -> w1881 mode=indexing
          tunnel: [w1888] -> w1880 mode=indexing
          tunnel: [w1887] -> w1879 mode=indexing
          tunnel: [w1886] -> w1878 mode=indexing
          i -> [w1893]
          (unwired) 0
          n77 = case shown="4" w1893 {
            tunnel: [FALSE TRUE TRUE TRUE FALSE] -> w1892
            tunnel: [TRUE FALSE FALSE FALSE TRUE] -> w1891
            tunnel: [TRUE FALSE FALSE FALSE TRUE] -> w1890
            tunnel: [TRUE FALSE FALSE FALSE TRUE] -> w1889
            tunnel: [TRUE FALSE FALSE FALSE TRUE] -> w1888
            tunnel: [TRUE FALSE FALSE FALSE TRUE] -> w1887
            tunnel: [FALSE TRUE TRUE TRUE FALSE] -> w1886
            frame 0, Default {
            }
            frame 1 {
            }
            frame 2 {
            }
            frame 3 {
            }
            frame 4 {
            }
          }
        }
      }
      frame "A" {
        n78 = for {
          N: 5 -> [_]
          tunnel: [w1943] -> w1935 mode=indexing
          tunnel: [w1942] -> w1934 mode=indexing
          tunnel: [w1941] -> w1933 mode=indexing
          tunnel: [w1940] -> w1932 mode=indexing
          tunnel: [w1939] -> w1931 mode=indexing
          tunnel: [w1938] -> w1930 mode=indexing
          tunnel: [w1937] -> w1929 mode=indexing
          i -> [w1944]
          (unwired) 0
          n79 = case shown="4" w1944 {
            tunnel: [FALSE TRUE TRUE TRUE FALSE] -> w1943
            tunnel: [TRUE FALSE FALSE FALSE TRUE] -> w1942
            tunnel: [TRUE FALSE FALSE FALSE TRUE] -> w1941
            tunnel: [TRUE TRUE TRUE TRUE TRUE] -> w1940
            tunnel: [TRUE FALSE FALSE FALSE TRUE] -> w1939
            tunnel: [TRUE FALSE FALSE FALSE TRUE] -> w1938
            tunnel: [TRUE FALSE FALSE FALSE TRUE] -> w1937
            frame 0, Default {
            }
            frame 1 {
            }
            frame 2 {
            }
            frame 3 {
            }
            frame 4 {
            }
          }
        }
      }
      frame "B" {
        n80 = for {
          N: 5 -> [_]
          tunnel: [w1994] -> w1986 mode=indexing
          tunnel: [w1993] -> w1985 mode=indexing
          tunnel: [w1992] -> w1984 mode=indexing
          tunnel: [w1991] -> w1983 mode=indexing
          tunnel: [w1990] -> w1982 mode=indexing
          tunnel: [w1989] -> w1981 mode=indexing
          tunnel: [w1988] -> w1980 mode=indexing
          i -> [w1995]
          (unwired) 0
          n81 = case shown="4" w1995 {
            tunnel: [TRUE TRUE TRUE TRUE FALSE] -> w1994
            tunnel: [TRUE FALSE FALSE FALSE TRUE] -> w1993
            tunnel: [TRUE FALSE FALSE FALSE TRUE] -> w1992
            tunnel: [TRUE TRUE TRUE TRUE FALSE] -> w1991
            tunnel: [TRUE FALSE FALSE FALSE TRUE] -> w1990
            tunnel: [TRUE FALSE FALSE FALSE TRUE] -> w1989
            tunnel: [TRUE TRUE TRUE TRUE FALSE] -> w1988
            frame 0, Default {
            }
            frame 1 {
            }
            frame 2 {
            }
            frame 3 {
            }
            frame 4 {
            }
          }
        }
      }
      frame "C" {
        n82 = for {
          N: 5 -> [_]
          tunnel: [w2045] -> w2037 mode=indexing
          tunnel: [w2044] -> w2036 mode=indexing
          tunnel: [w2043] -> w2035 mode=indexing
          tunnel: [w2042] -> w2034 mode=indexing
          tunnel: [w2041] -> w2033 mode=indexing
          tunnel: [w2040] -> w2032 mode=indexing
          tunnel: [w2039] -> w2031 mode=indexing
          i -> [w2046]
          (unwired) 0
          n83 = case shown="4" w2046 {
            tunnel: [FALSE TRUE TRUE TRUE FALSE] -> w2045
            tunnel: [TRUE FALSE FALSE FALSE TRUE] -> w2044
            tunnel: [TRUE FALSE FALSE FALSE FALSE] -> w2043
            tunnel: [TRUE FALSE FALSE FALSE FALSE] -> w2042
            tunnel: [TRUE FALSE FALSE FALSE FALSE] -> w2041
            tunnel: [TRUE FALSE FALSE FALSE TRUE] -> w2040
            tunnel: [FALSE TRUE TRUE TRUE FALSE] -> w2039
            frame 0, Default {
            }
            frame 1 {
            }
            frame 2 {
            }
            frame 3 {
            }
            frame 4 {
            }
          }
        }
      }
      frame "D" {
        n84 = for {
          N: 5 -> [_]
          tunnel: [w2096] -> w2088 mode=indexing
          tunnel: [w2095] -> w2087 mode=indexing
          tunnel: [w2094] -> w2086 mode=indexing
          tunnel: [w2093] -> w2085 mode=indexing
          tunnel: [w2092] -> w2084 mode=indexing
          tunnel: [w2091] -> w2083 mode=indexing
          tunnel: [w2090] -> w2082 mode=indexing
          i -> [w2097]
          (unwired) 0
          n85 = case shown="4" w2097 {
            tunnel: [TRUE TRUE TRUE TRUE FALSE] -> w2096
            tunnel: [TRUE FALSE FALSE FALSE TRUE] -> w2095
            tunnel: [TRUE FALSE FALSE FALSE TRUE] -> w2094
            tunnel: [TRUE FALSE FALSE FALSE TRUE] -> w2093
            tunnel: [TRUE FALSE FALSE FALSE TRUE] -> w2092
            tunnel: [TRUE FALSE FALSE FALSE TRUE] -> w2091
            tunnel: [TRUE TRUE TRUE TRUE FALSE] -> w2090
            frame 0, Default {
            }
            frame 1 {
            }
            frame 2 {
            }
            frame 3 {
            }
            frame 4 {
            }
          }
        }
      }
      frame "E" {
        n86 = for {
          N: 5 -> [_]
          tunnel: [w2147] -> w2139 mode=indexing
          tunnel: [w2146] -> w2138 mode=indexing
          tunnel: [w2145] -> w2137 mode=indexing
          tunnel: [w2144] -> w2136 mode=indexing
          tunnel: [w2143] -> w2135 mode=indexing
          tunnel: [w2142] -> w2134 mode=indexing
          tunnel: [w2141] -> w2133 mode=indexing
          i -> [w2148]
          (unwired) 0
          n87 = case shown="0, Default" w2148 {
            tunnel: [TRUE TRUE TRUE TRUE TRUE] -> w2147
            tunnel: [TRUE FALSE FALSE FALSE FALSE] -> w2146
            tunnel: [TRUE FALSE FALSE FALSE FALSE] -> w2145
            tunnel: [TRUE TRUE TRUE TRUE FALSE] -> w2144
            tunnel: [TRUE FALSE FALSE FALSE FALSE] -> w2143
            tunnel: [TRUE FALSE FALSE FALSE FALSE] -> w2142
            tunnel: [TRUE TRUE TRUE TRUE TRUE] -> w2141
            frame 0, Default {
            }
            frame 1 {
            }
            frame 2 {
            }
            frame 3 {
            }
            frame 4 {
            }
          }
        }
      }
      frame "F" {
        n88 = for {
          N: 5 -> [_]
          tunnel: [w2198] -> w2190 mode=indexing
          tunnel: [w2197] -> w2189 mode=indexing
          tunnel: [w2196] -> w2188 mode=indexing
          tunnel: [w2195] -> w2187 mode=indexing
          tunnel: [w2194] -> w2186 mode=indexing
          tunnel: [w2193] -> w2185 mode=indexing
          tunnel: [w2192] -> w2184 mode=indexing
          i -> [w2199]
          (unwired) 0
          n89 = case shown="0, Default" w2199 {
            tunnel: [TRUE TRUE TRUE TRUE TRUE] -> w2198
            tunnel: [TRUE FALSE FALSE FALSE FALSE] -> w2197
            tunnel: [TRUE FALSE FALSE FALSE FALSE] -> w2196
            tunnel: [TRUE TRUE TRUE TRUE FALSE] -> w2195
            tunnel: [TRUE FALSE FALSE FALSE FALSE] -> w2194
            tunnel: [TRUE FALSE FALSE FALSE FALSE] -> w2193
            tunnel: [TRUE FALSE FALSE FALSE FALSE] -> w2192
            frame 0, Default {
            }
            frame 1 {
            }
            frame 2 {
            }
            frame 3 {
            }
            frame 4 {
            }
          }
        }
      }
      frame "G" {
        n90 = for {
          N: 5 -> [_]
          tunnel: [w2249] -> w2241 mode=indexing
          tunnel: [w2248] -> w2240 mode=indexing
          tunnel: [w2247] -> w2239 mode=indexing
          tunnel: [w2246] -> w2238 mode=indexing
          tunnel: [w2245] -> w2237 mode=indexing
          tunnel: [w2244] -> w2236 mode=indexing
          tunnel: [w2243] -> w2235 mode=indexing
          i -> [w2250]
          (unwired) 0
          n91 = case shown="0, Default" w2250 {
            tunnel: [FALSE TRUE TRUE TRUE TRUE] -> w2249
            tunnel: [TRUE FALSE FALSE FALSE FALSE] -> w2248
            tunnel: [TRUE FALSE FALSE FALSE FALSE] -> w2247
            tunnel: [TRUE FALSE FALSE TRUE TRUE] -> w2246
            tunnel: [TRUE FALSE FALSE FALSE TRUE] -> w2245
            tunnel: [TRUE FALSE FALSE FALSE TRUE] -> w2244
            tunnel: [FALSE TRUE TRUE TRUE FALSE] -> w2243
            frame 0, Default {
            }
            frame 1 {
            }
            frame 2 {
            }
            frame 3 {
            }
            frame 4 {
            }
          }
        }
      }
      frame "H" {
        n92 = for {
          N: 5 -> [_]
          tunnel: [w2300] -> w2292 mode=indexing
          tunnel: [w2299] -> w2291 mode=indexing
          tunnel: [w2298] -> w2290 mode=indexing
          tunnel: [w2297] -> w2289 mode=indexing
          tunnel: [w2296] -> w2288 mode=indexing
          tunnel: [w2295] -> w2287 mode=indexing
          tunnel: [w2294] -> w2286 mode=indexing
          i -> [w2301]
          (unwired) 0
          n93 = case shown="4" w2301 {
            tunnel: [TRUE FALSE FALSE FALSE TRUE] -> w2300
            tunnel: [TRUE FALSE FALSE FALSE TRUE] -> w2299
            tunnel: [TRUE FALSE FALSE FALSE TRUE] -> w2298
            tunnel: [TRUE TRUE TRUE TRUE TRUE] -> w2297
            tunnel: [TRUE FALSE FALSE FALSE TRUE] -> w2296
            tunnel: [TRUE FALSE FALSE FALSE TRUE] -> w2295
            tunnel: [TRUE FALSE FALSE FALSE TRUE] -> w2294
            frame 0, Default {
            }
            frame 1 {
            }
            frame 2 {
            }
            frame 3 {
            }
            frame 4 {
            }
          }
        }
      }
      frame "I" {
        n94 = for {
          N: 5 -> [_]
          tunnel: [w2351] -> w2343 mode=indexing
          tunnel: [w2350] -> w2342 mode=indexing
          tunnel: [w2349] -> w2341 mode=indexing
          tunnel: [w2348] -> w2340 mode=indexing
          tunnel: [w2347] -> w2339 mode=indexing
          tunnel: [w2346] -> w2338 mode=indexing
          tunnel: [w2345] -> w2337 mode=indexing
          i -> [w2352]
          (unwired) 0
          n95 = case shown="0, Default" w2352 {
            tunnel: [TRUE TRUE TRUE TRUE TRUE] -> w2351
            tunnel: [FALSE FALSE TRUE FALSE FALSE] -> w2350
            tunnel: [FALSE FALSE TRUE FALSE FALSE] -> w2349
            tunnel: [FALSE FALSE TRUE FALSE FALSE] -> w2348
            tunnel: [FALSE FALSE TRUE FALSE FALSE] -> w2347
            tunnel: [FALSE FALSE TRUE FALSE FALSE] -> w2346
            tunnel: [TRUE TRUE TRUE TRUE TRUE] -> w2345
            frame 0, Default {
            }
            frame 1 {
            }
            frame 2 {
            }
            frame 3 {
            }
            frame 4 {
            }
          }
        }
      }
      frame "J" {
        n96 = for {
          N: 5 -> [_]
          tunnel: [w2402] -> w2394 mode=indexing
          tunnel: [w2401] -> w2393 mode=indexing
          tunnel: [w2400] -> w2392 mode=indexing
          tunnel: [w2399] -> w2391 mode=indexing
          tunnel: [w2398] -> w2390 mode=indexing
          tunnel: [w2397] -> w2389 mode=indexing
          tunnel: [w2396] -> w2388 mode=indexing
          i -> [w2403]
          (unwired) 0
          n97 = case shown="0, Default" w2403 {
            tunnel: [TRUE TRUE TRUE TRUE TRUE] -> w2402
            tunnel: [FALSE FALSE TRUE FALSE FALSE] -> w2401
            tunnel: [FALSE FALSE TRUE FALSE FALSE] -> w2400
            tunnel: [FALSE FALSE TRUE FALSE FALSE] -> w2399
            tunnel: [FALSE FALSE TRUE FALSE FALSE] -> w2398
            tunnel: [TRUE FALSE TRUE FALSE FALSE] -> w2397
            tunnel: [FALSE TRUE TRUE FALSE FALSE] -> w2396
            frame 0, Default {
            }
            frame 1 {
            }
            frame 2 {
            }
            frame 3 {
            }
            frame 4 {
            }
          }
        }
      }
      frame "K" {
        n98 = for {
          N: 5 -> [_]
          tunnel: [w2453] -> w2445 mode=indexing
          tunnel: [w2452] -> w2444 mode=indexing
          tunnel: [w2451] -> w2443 mode=indexing
          tunnel: [w2450] -> w2442 mode=indexing
          tunnel: [w2449] -> w2441 mode=indexing
          tunnel: [w2448] -> w2440 mode=indexing
          tunnel: [w2447] -> w2439 mode=indexing
          i -> [w2454]
          (unwired) 0
          n99 = case shown="4" w2454 {
            tunnel: [TRUE FALSE FALSE FALSE TRUE] -> w2453
            tunnel: [TRUE FALSE FALSE TRUE FALSE] -> w2452
            tunnel: [TRUE FALSE TRUE FALSE FALSE] -> w2451
            tunnel: [TRUE TRUE FALSE FALSE FALSE] -> w2450
            tunnel: [TRUE FALSE TRUE FALSE FALSE] -> w2449
            tunnel: [TRUE FALSE FALSE TRUE FALSE] -> w2448
            tunnel: [TRUE FALSE FALSE FALSE TRUE] -> w2447
            frame 0, Default {
            }
            frame 1 {
            }
            frame 2 {
            }
            frame 3 {
            }
            frame 4 {
            }
          }
        }
      }
      frame "L" {
        n100 = for {
          N: 5 -> [_]
          tunnel: [w2504] -> w2496 mode=indexing
          tunnel: [w2503] -> w2495 mode=indexing
          tunnel: [w2502] -> w2494 mode=indexing
          tunnel: [w2501] -> w2493 mode=indexing
          tunnel: [w2500] -> w2492 mode=indexing
          tunnel: [w2499] -> w2491 mode=indexing
          tunnel: [w2498] -> w2490 mode=indexing
          i -> [w2505]
          (unwired) 0
          n101 = case shown="0, Default" w2505 {
            tunnel: [TRUE FALSE FALSE FALSE FALSE] -> w2504
            tunnel: [TRUE FALSE FALSE FALSE FALSE] -> w2503
            tunnel: [TRUE FALSE FALSE FALSE FALSE] -> w2502
            tunnel: [TRUE FALSE FALSE FALSE FALSE] -> w2501
            tunnel: [TRUE FALSE FALSE FALSE FALSE] -> w2500
            tunnel: [TRUE FALSE FALSE FALSE FALSE] -> w2499
            tunnel: [TRUE TRUE TRUE TRUE TRUE] -> w2498
            frame 0, Default {
            }
            frame 1 {
            }
            frame 2 {
            }
            frame 3 {
            }
            frame 4 {
            }
          }
        }
      }
      frame "M" {
        n102 = for {
          N: 5 -> [_]
          tunnel: [w2555] -> w2547 mode=indexing
          tunnel: [w2554] -> w2546 mode=indexing
          tunnel: [w2553] -> w2545 mode=indexing
          tunnel: [w2552] -> w2544 mode=indexing
          tunnel: [w2551] -> w2543 mode=indexing
          tunnel: [w2550] -> w2542 mode=indexing
          tunnel: [w2549] -> w2541 mode=indexing
          i -> [w2556]
          (unwired) 0
          n103 = case shown="4" w2556 {
            tunnel: [TRUE FALSE FALSE FALSE TRUE] -> w2555
            tunnel: [TRUE TRUE FALSE TRUE TRUE] -> w2554
            tunnel: [TRUE FALSE TRUE FALSE TRUE] -> w2553
            tunnel: [TRUE FALSE FALSE FALSE TRUE] -> w2552
            tunnel: [TRUE FALSE FALSE FALSE TRUE] -> w2551
            tunnel: [TRUE FALSE FALSE FALSE TRUE] -> w2550
            tunnel: [TRUE FALSE FALSE FALSE TRUE] -> w2549
            frame 0, Default {
            }
            frame 1 {
            }
            frame 2 {
            }
            frame 3 {
            }
            frame 4 {
            }
          }
        }
      }
      frame "N" {
        n104 = for {
          N: 5 -> [_]
          tunnel: [w2606] -> w2598 mode=indexing
          tunnel: [w2605] -> w2597 mode=indexing
          tunnel: [w2604] -> w2596 mode=indexing
          tunnel: [w2603] -> w2595 mode=indexing
          tunnel: [w2602] -> w2594 mode=indexing
          tunnel: [w2601] -> w2593 mode=indexing
          tunnel: [w2600] -> w2592 mode=indexing
          i -> [w2607]
          (unwired) 0
          n105 = case shown="0, Default" w2607 {
            tunnel: [TRUE FALSE FALSE FALSE TRUE] -> w2606
            tunnel: [TRUE TRUE FALSE FALSE TRUE] -> w2605
            tunnel: [TRUE TRUE TRUE FALSE TRUE] -> w2604
            tunnel: [TRUE TRUE TRUE TRUE TRUE] -> w2603
            tunnel: [TRUE FALSE TRUE TRUE TRUE] -> w2602
            tunnel: [TRUE FALSE FALSE TRUE TRUE] -> w2601
            tunnel: [TRUE FALSE FALSE FALSE TRUE] -> w2600
            frame 0, Default {
            }
            frame 1 {
            }
            frame 2 {
            }
            frame 3 {
            }
            frame 4 {
            }
          }
        }
      }
      frame "O" {
        n106 = for {
          N: 5 -> [_]
          tunnel: [w2657] -> w2649 mode=indexing
          tunnel: [w2656] -> w2648 mode=indexing
          tunnel: [w2655] -> w2647 mode=indexing
          tunnel: [w2654] -> w2646 mode=indexing
          tunnel: [w2653] -> w2645 mode=indexing
          tunnel: [w2652] -> w2644 mode=indexing
          tunnel: [w2651] -> w2643 mode=indexing
          i -> [w2658]
          (unwired) 0
          n107 = case shown="0, Default" w2658 {
            tunnel: [FALSE TRUE TRUE TRUE FALSE] -> w2657
            tunnel: [TRUE FALSE FALSE FALSE TRUE] -> w2656
            tunnel: [TRUE FALSE FALSE FALSE TRUE] -> w2655
            tunnel: [TRUE FALSE FALSE FALSE TRUE] -> w2654
            tunnel: [TRUE FALSE FALSE FALSE TRUE] -> w2653
            tunnel: [TRUE FALSE FALSE FALSE TRUE] -> w2652
            tunnel: [FALSE TRUE TRUE TRUE FALSE] -> w2651
            frame 0, Default {
            }
            frame 1 {
            }
            frame 2 {
            }
            frame 3 {
            }
            frame 4 {
            }
          }
        }
      }
      frame "P" {
        n108 = for {
          N: 5 -> [_]
          tunnel: [w2708] -> w2700 mode=indexing
          tunnel: [w2707] -> w2699 mode=indexing
          tunnel: [w2706] -> w2698 mode=indexing
          tunnel: [w2705] -> w2697 mode=indexing
          tunnel: [w2704] -> w2696 mode=indexing
          tunnel: [w2703] -> w2695 mode=indexing
          tunnel: [w2702] -> w2694 mode=indexing
          i -> [w2709]
          (unwired) 0
          n109 = case shown="0, Default" w2709 {
            tunnel: [TRUE TRUE TRUE TRUE FALSE] -> w2708
            tunnel: [TRUE FALSE FALSE FALSE TRUE] -> w2707
            tunnel: [TRUE FALSE FALSE FALSE TRUE] -> w2706
            tunnel: [TRUE TRUE TRUE TRUE FALSE] -> w2705
            tunnel: [TRUE FALSE FALSE FALSE FALSE] -> w2704
            tunnel: [TRUE FALSE FALSE FALSE FALSE] -> w2703
            tunnel: [TRUE FALSE FALSE FALSE FALSE] -> w2702
            frame 0, Default {
            }
            frame 1 {
            }
            frame 2 {
            }
            frame 3 {
            }
            frame 4 {
            }
          }
        }
      }
      frame "Q" {
        n110 = for {
          N: 5 -> [_]
          tunnel: [w2759] -> w2751 mode=indexing
          tunnel: [w2758] -> w2750 mode=indexing
          tunnel: [w2757] -> w2749 mode=indexing
          tunnel: [w2756] -> w2748 mode=indexing
          tunnel: [w2755] -> w2747 mode=indexing
          tunnel: [w2754] -> w2746 mode=indexing
          tunnel: [w2753] -> w2745 mode=indexing
          i -> [w2760]
          (unwired) 0
          n111 = case shown="4" w2760 {
            tunnel: [FALSE TRUE TRUE TRUE FALSE] -> w2759
            tunnel: [TRUE FALSE FALSE FALSE TRUE] -> w2758
            tunnel: [TRUE FALSE FALSE FALSE TRUE] -> w2757
            tunnel: [TRUE FALSE FALSE FALSE TRUE] -> w2756
            tunnel: [TRUE FALSE FALSE FALSE TRUE] -> w2755
            tunnel: [TRUE FALSE FALSE TRUE TRUE] -> w2754
            tunnel: [FALSE TRUE TRUE TRUE TRUE] -> w2753
            frame 0, Default {
            }
            frame 1 {
            }
            frame 2 {
            }
            frame 3 {
            }
            frame 4 {
            }
          }
        }
      }
      frame "R" {
        n112 = for {
          N: 5 -> [_]
          tunnel: [w2810] -> w2802 mode=indexing
          tunnel: [w2809] -> w2801 mode=indexing
          tunnel: [w2808] -> w2800 mode=indexing
          tunnel: [w2807] -> w2799 mode=indexing
          tunnel: [w2806] -> w2798 mode=indexing
          tunnel: [w2805] -> w2797 mode=indexing
          tunnel: [w2804] -> w2796 mode=indexing
          i -> [w2811]
          (unwired) 0
          n113 = case shown="2" w2811 {
            tunnel: [TRUE TRUE TRUE TRUE FALSE] -> w2810
            tunnel: [TRUE FALSE FALSE FALSE TRUE] -> w2809
            tunnel: [TRUE FALSE FALSE FALSE TRUE] -> w2808
            tunnel: [TRUE TRUE TRUE TRUE FALSE] -> w2807
            tunnel: [TRUE TRUE TRUE FALSE FALSE] -> w2806
            tunnel: [TRUE FALSE TRUE TRUE FALSE] -> w2805
            tunnel: [TRUE FALSE FALSE TRUE TRUE] -> w2804
            frame 0, Default {
            }
            frame 1 {
            }
            frame 2 {
            }
            frame 3 {
            }
            frame 4 {
            }
          }
        }
      }
      frame "S" {
        n114 = for {
          N: 5 -> [_]
          tunnel: [w2861] -> w2853 mode=indexing
          tunnel: [w2860] -> w2852 mode=indexing
          tunnel: [w2859] -> w2851 mode=indexing
          tunnel: [w2858] -> w2850 mode=indexing
          tunnel: [w2857] -> w2849 mode=indexing
          tunnel: [w2856] -> w2848 mode=indexing
          tunnel: [w2855] -> w2847 mode=indexing
          i -> [w2862]
          (unwired) 0
          n115 = case shown="0, Default" w2862 {
            tunnel: [FALSE TRUE TRUE TRUE FALSE] -> w2861
            tunnel: [TRUE FALSE FALSE FALSE TRUE] -> w2860
            tunnel: [TRUE FALSE FALSE FALSE FALSE] -> w2859
            tunnel: [TRUE TRUE TRUE TRUE TRUE] -> w2858
            tunnel: [FALSE FALSE FALSE FALSE TRUE] -> w2857
            tunnel: [TRUE FALSE FALSE FALSE TRUE] -> w2856
            tunnel: [FALSE TRUE TRUE TRUE FALSE] -> w2855
            frame 0, Default {
            }
            frame 1 {
            }
            frame 2 {
            }
            frame 3 {
            }
            frame 4 {
            }
          }
        }
      }
      frame "T" {
        n116 = for {
          N: 5 -> [_]
          tunnel: [w2912] -> w2904 mode=indexing
          tunnel: [w2911] -> w2903 mode=indexing
          tunnel: [w2910] -> w2902 mode=indexing
          tunnel: [w2909] -> w2901 mode=indexing
          tunnel: [w2908] -> w2900 mode=indexing
          tunnel: [w2907] -> w2899 mode=indexing
          tunnel: [w2906] -> w2898 mode=indexing
          i -> [w2913]
          (unwired) 0
          n117 = case shown="0, Default" w2913 {
            tunnel: [TRUE TRUE TRUE TRUE TRUE] -> w2912
            tunnel: [FALSE FALSE TRUE FALSE FALSE] -> w2911
            tunnel: [FALSE FALSE TRUE FALSE FALSE] -> w2910
            tunnel: [FALSE FALSE TRUE FALSE FALSE] -> w2909
            tunnel: [FALSE FALSE TRUE FALSE FALSE] -> w2908
            tunnel: [FALSE FALSE TRUE FALSE FALSE] -> w2907
            tunnel: [FALSE FALSE TRUE FALSE FALSE] -> w2906
            frame 0, Default {
            }
            frame 1 {
            }
            frame 2 {
            }
            frame 3 {
            }
            frame 4 {
            }
          }
        }
      }
      frame "U" {
        n118 = for {
          N: 5 -> [_]
          tunnel: [w2963] -> w2955 mode=indexing
          tunnel: [w2962] -> w2954 mode=indexing
          tunnel: [w2961] -> w2953 mode=indexing
          tunnel: [w2960] -> w2952 mode=indexing
          tunnel: [w2959] -> w2951 mode=indexing
          tunnel: [w2958] -> w2950 mode=indexing
          tunnel: [w2957] -> w2949 mode=indexing
          i -> [w2964]
          (unwired) 0
          n119 = case shown="0, Default" w2964 {
            tunnel: [TRUE FALSE FALSE FALSE TRUE] -> w2963
            tunnel: [TRUE FALSE FALSE FALSE TRUE] -> w2962
            tunnel: [TRUE FALSE FALSE FALSE TRUE] -> w2961
            tunnel: [TRUE FALSE FALSE FALSE TRUE] -> w2960
            tunnel: [TRUE FALSE FALSE FALSE TRUE] -> w2959
            tunnel: [TRUE FALSE FALSE FALSE TRUE] -> w2958
            tunnel: [FALSE TRUE TRUE TRUE FALSE] -> w2957
            frame 0, Default {
            }
            frame 1 {
            }
            frame 2 {
            }
            frame 3 {
            }
            frame 4 {
            }
          }
        }
      }
      frame "V" {
        n120 = for {
          N: 5 -> [_]
          tunnel: [w3014] -> w3006 mode=indexing
          tunnel: [w3013] -> w3005 mode=indexing
          tunnel: [w3012] -> w3004 mode=indexing
          tunnel: [w3011] -> w3003 mode=indexing
          tunnel: [w3010] -> w3002 mode=indexing
          tunnel: [w3009] -> w3001 mode=indexing
          tunnel: [w3008] -> w3000 mode=indexing
          i -> [w3015]
          (unwired) 0
          n121 = case shown="0, Default" w3015 {
            tunnel: [TRUE FALSE FALSE FALSE TRUE] -> w3014
            tunnel: [TRUE FALSE FALSE FALSE TRUE] -> w3013
            tunnel: [TRUE FALSE FALSE FALSE TRUE] -> w3012
            tunnel: [TRUE FALSE FALSE FALSE TRUE] -> w3011
            tunnel: [TRUE FALSE FALSE FALSE TRUE] -> w3010
            tunnel: [FALSE TRUE FALSE TRUE FALSE] -> w3009
            tunnel: [FALSE FALSE TRUE FALSE FALSE] -> w3008
            frame 0, Default {
            }
            frame 1 {
            }
            frame 2 {
            }
            frame 3 {
            }
            frame 4 {
            }
          }
        }
      }
      frame "W" {
        n122 = for {
          N: 5 -> [_]
          tunnel: [w3065] -> w3057 mode=indexing
          tunnel: [w3064] -> w3056 mode=indexing
          tunnel: [w3063] -> w3055 mode=indexing
          tunnel: [w3062] -> w3054 mode=indexing
          tunnel: [w3061] -> w3053 mode=indexing
          tunnel: [w3060] -> w3052 mode=indexing
          tunnel: [w3059] -> w3051 mode=indexing
          i -> [w3066]
          (unwired) 0
          n123 = case shown="0, Default" w3066 {
            tunnel: [TRUE FALSE FALSE FALSE TRUE] -> w3065
            tunnel: [TRUE FALSE FALSE FALSE TRUE] -> w3064
            tunnel: [TRUE FALSE FALSE FALSE TRUE] -> w3063
            tunnel: [TRUE FALSE TRUE FALSE TRUE] -> w3062
            tunnel: [TRUE FALSE TRUE FALSE TRUE] -> w3061
            tunnel: [TRUE TRUE FALSE TRUE TRUE] -> w3060
            tunnel: [TRUE FALSE FALSE FALSE TRUE] -> w3059
            frame 0, Default {
            }
            frame 1 {
            }
            frame 2 {
            }
            frame 3 {
            }
            frame 4 {
            }
          }
        }
      }
      frame "X" {
        n124 = for {
          N: 5 -> [_]
          tunnel: [w3116] -> w3108 mode=indexing
          tunnel: [w3115] -> w3107 mode=indexing
          tunnel: [w3114] -> w3106 mode=indexing
          tunnel: [w3113] -> w3105 mode=indexing
          tunnel: [w3112] -> w3104 mode=indexing
          tunnel: [w3111] -> w3103 mode=indexing
          tunnel: [w3110] -> w3102 mode=indexing
          i -> [w3117]
          (unwired) 0
          n125 = case shown="0, Default" w3117 {
            tunnel: [TRUE TRUE FALSE TRUE TRUE] -> w3116
            tunnel: [TRUE TRUE FALSE TRUE TRUE] -> w3115
            tunnel: [FALSE TRUE FALSE TRUE FALSE] -> w3114
            tunnel: [FALSE FALSE TRUE FALSE FALSE] -> w3113
            tunnel: [FALSE TRUE FALSE TRUE FALSE] -> w3112
            tunnel: [TRUE TRUE FALSE TRUE TRUE] -> w3111
            tunnel: [TRUE TRUE FALSE TRUE TRUE] -> w3110
            frame 0, Default {
            }
            frame 1 {
            }
            frame 2 {
            }
            frame 3 {
            }
            frame 4 {
            }
          }
        }
      }
      frame "Y" {
        n126 = for {
          N: 5 -> [_]
          tunnel: [w3167] -> w3159 mode=indexing
          tunnel: [w3166] -> w3158 mode=indexing
          tunnel: [w3165] -> w3157 mode=indexing
          tunnel: [w3164] -> w3156 mode=indexing
          tunnel: [w3163] -> w3155 mode=indexing
          tunnel: [w3162] -> w3154 mode=indexing
          tunnel: [w3161] -> w3153 mode=indexing
          i -> [w3168]
          (unwired) 0
          n127 = case shown="1" w3168 {
            tunnel: [TRUE FALSE FALSE FALSE TRUE] -> w3167
            tunnel: [TRUE FALSE FALSE FALSE TRUE] -> w3166
            tunnel: [TRUE FALSE FALSE FALSE TRUE] -> w3165
            tunnel: [FALSE TRUE TRUE TRUE FALSE] -> w3164
            tunnel: [FALSE FALSE TRUE FALSE FALSE] -> w3163
            tunnel: [FALSE FALSE TRUE FALSE FALSE] -> w3162
            tunnel: [FALSE FALSE TRUE FALSE FALSE] -> w3161
            frame 0, Default {
            }
            frame 1 {
            }
            frame 2 {
            }
            frame 3 {
            }
            frame 4 {
            }
          }
        }
      }
      frame "Z" {
        n128 = for {
          N: 5 -> [_]
          tunnel: [w3218] -> w3210 mode=indexing
          tunnel: [w3217] -> w3209 mode=indexing
          tunnel: [w3216] -> w3208 mode=indexing
          tunnel: [w3215] -> w3207 mode=indexing
          tunnel: [w3214] -> w3206 mode=indexing
          tunnel: [w3213] -> w3205 mode=indexing
          tunnel: [w3212] -> w3204 mode=indexing
          i -> [w3219]
          (unwired) 0
          n129 = case shown="1" w3219 {
            tunnel: [TRUE TRUE TRUE TRUE TRUE] -> w3218
            tunnel: [FALSE FALSE FALSE FALSE TRUE] -> w3217
            tunnel: [FALSE FALSE FALSE TRUE FALSE] -> w3216
            tunnel: [FALSE FALSE TRUE FALSE FALSE] -> w3215
            tunnel: [FALSE TRUE FALSE FALSE FALSE] -> w3214
            tunnel: [TRUE FALSE FALSE FALSE FALSE] -> w3213
            tunnel: [TRUE TRUE TRUE TRUE TRUE] -> w3212
            frame 0, Default {
            }
            frame 1 {
            }
            frame 2 {
            }
            frame 3 {
            }
            frame 4 {
            }
          }
        }
      }
    }
    "Array 1" <- w18
    "Array 2" <- w17
    "Array 3" <- w29
    "Array 4" <- w24
    "Array 5" <- w16
    "Array 6" <- w7
    "Array 7" <- w6
    n130 = Boolean To (0,1)(Boolean=w18) -> (0, 1=w40:i16[])
    n131 = Boolean To (0,1)(Boolean=w29) -> (0, 1=w33:i16[])
    n132 = Boolean To (0,1)(Boolean=w17) -> (0, 1=w34:i16[])
    n133 = Boolean Array To Number(Boolean array=w17) -> ()  [unwired: 1 out]
    n134 = Boolean To (0,1)(Boolean=w16) -> (0, 1=w23:i16[])
    n135 = Boolean To (0,1)(Boolean=w7) -> (0, 1=w15:i16[])
    n136 = Boolean To (0,1)(Boolean=w6) -> (0, 1=w11:i16[])
    n137 = Boolean Array To Number(Boolean array=w18) -> ()  [unwired: 1 out]
    n138 = Boolean To (0,1)(Boolean=w24) -> (0, 1=w28:i16[])
    n139 = Number To Decimal String(number=w40) -> (decimal integer string=w39:string[])  [unwired: 1 in]
    n140 = Number To Decimal String(number=w33) -> (decimal integer string=w32:string[])  [unwired: 1 in]
    n141 = Number To Decimal String(number=w34) -> (decimal integer string=w35:string[])  [unwired: 1 in]
    n142 = Number To Decimal String(number=w28) -> (decimal integer string=w27:string[])  [unwired: 1 in]
    n143 = Number To Decimal String(number=w23) -> (decimal integer string=w22:string[])  [unwired: 1 in]
    n144 = Number To Decimal String(number=w15) -> (decimal integer string=w14:string[])  [unwired: 1 in]
    n145 = Number To Decimal String(number=w11) -> (decimal integer string=w10:string[])  [unwired: 1 in]
    n146 = Concatenate Strings(w39) -> (w38:string)
    n147 = Concatenate Strings(w32) -> (w31:string)
    n148 = Concatenate Strings(w35) -> (w19:string)
    n149 = Concatenate Strings(w27) -> (w26:string)
    n150 = Concatenate Strings(w22) -> (w21:string)
    n151 = Concatenate Strings(w14) -> (w13:string)
    n152 = Concatenate Strings(w10) -> (w9:string)
    n153 = String To Byte Array(string=w38) -> (unsigned byte array=w37:u8[])
    n154 = String To Byte Array(string=w31) -> (unsigned byte array=w30:u8[])
    n155 = String To Byte Array(string=w19) -> (unsigned byte array=w36:u8[])
    n156 = String To Byte Array(string=w26) -> (unsigned byte array=w25:u8[])
    n157 = String To Byte Array(string=w21) -> (unsigned byte array=w20:u8[])
    n158 = String To Byte Array(string=w13) -> (unsigned byte array=w12:u8[])
    n159 = String To Byte Array(string=w9) -> (unsigned byte array=w8:u8[])
    n160 = for {
      tunnel: w37 -> [w90] mode=indexing
      tunnel: w5 -> [w86]
      n161 = Build Array(w90) -> (w87:u8[])
      n162 = Byte Array To String(unsigned byte array=w87) -> (string=w89:string)
      n163 = case shown="\"1\"" w89 {
        tunnel: [FALSE TRUE] -> w88
        frame "0", Default {
        }
        frame "1" {
        }
      }
      "Boolean" <- w88
      n164 = Wait (ms)(milliseconds to wait=w86) -> ()  [unwired: 1 out]
    }
    n165 = for {
      tunnel: w30 -> [w76] mode=indexing
      tunnel: w4 -> [w72]
      n166 = Build Array(w76) -> (w73:u8[])
      n167 = Byte Array To String(unsigned byte array=w73) -> (string=w75:string)
      n168 = case shown="\"1\"" w75 {
        tunnel: [FALSE TRUE] -> w74
        frame "0", Default {
        }
        frame "1" {
        }
      }
      "Boolean 3" <- w74
      n169 = Wait (ms)(milliseconds to wait=w72) -> ()  [unwired: 1 out]
    }
    n170 = for {
      tunnel: w36 -> [w83] mode=indexing
      tunnel: w4 -> [w79]
      n171 = Build Array(w83) -> (w80:u8[])
      n172 = Byte Array To String(unsigned byte array=w80) -> (string=w82:string)
      n173 = case shown="\"1\"" w82 {
        tunnel: [FALSE TRUE] -> w81
        frame "0", Default {
        }
        frame "1" {
        }
      }
      "Boolean 2" <- w81
      n174 = Wait (ms)(milliseconds to wait=w79) -> ()  [unwired: 1 out]
    }
    n175 = for {
      tunnel: w25 -> [w69] mode=indexing
      tunnel: w4 -> [w65]
      n176 = Build Array(w69) -> (w66:u8[])
      n177 = Byte Array To String(unsigned byte array=w66) -> (string=w68:string)
      n178 = case shown="\"1\"" w68 {
        tunnel: [FALSE TRUE] -> w67
        frame "0", Default {
        }
        frame "1" {
        }
      }
      "Boolean 4" <- w67
      n179 = Wait (ms)(milliseconds to wait=w65) -> ()  [unwired: 1 out]
    }
    n180 = for {
      tunnel: w20 -> [w62] mode=indexing
      tunnel: w4 -> [w58]
      n181 = Build Array(w62) -> (w59:u8[])
      n182 = Byte Array To String(unsigned byte array=w59) -> (string=w61:string)
      n183 = case shown="\"1\"" w61 {
        tunnel: [FALSE TRUE] -> w60
        frame "0", Default {
        }
        frame "1" {
        }
      }
      "Boolean 5" <- w60
      n184 = Wait (ms)(milliseconds to wait=w58) -> ()  [unwired: 1 out]
    }
    n185 = for {
      tunnel: w12 -> [w55] mode=indexing
      tunnel: w4 -> [w51]
      n186 = Build Array(w55) -> (w52:u8[])
      n187 = Byte Array To String(unsigned byte array=w52) -> (string=w54:string)
      n188 = case shown="\"1\"" w54 {
        tunnel: [FALSE TRUE] -> w53
        frame "0", Default {
        }
        frame "1" {
        }
      }
      "Boolean 6" <- w53
      n189 = Wait (ms)(milliseconds to wait=w51) -> ()  [unwired: 1 out]
    }
    n190 = for {
      tunnel: w8 -> [w48] mode=indexing
      tunnel: w4 -> [w44]
      n191 = Build Array(w48) -> (w45:u8[])
      n192 = Byte Array To String(unsigned byte array=w45) -> (string=w47:string)
      n193 = case shown="\"1\"" w47 {
        tunnel: [FALSE TRUE] -> w46
        frame "0", Default {
        }
        frame "1" {
        }
      }
      "Boolean 7" <- w46
      n194 = Wait (ms)(milliseconds to wait=w44) -> ()  [unwired: 1 out]
    }
  }
